vi "Lab03_Correct.vi"() -> ()   [LabVIEW 2022 SP3]
uses:
  <vilib>/numeric/Random Number (Range) DBL.vi
panel:
  out "Phase":dbl
  out "Sum of Differences Graph":cluster{dbl[], dbl[]}(graph)
  out "Sum of Difference Array":dbl[](array[numeric])
  out "Noisy Signal":dbl[][](graph)
  in  "# of Periods":dbl
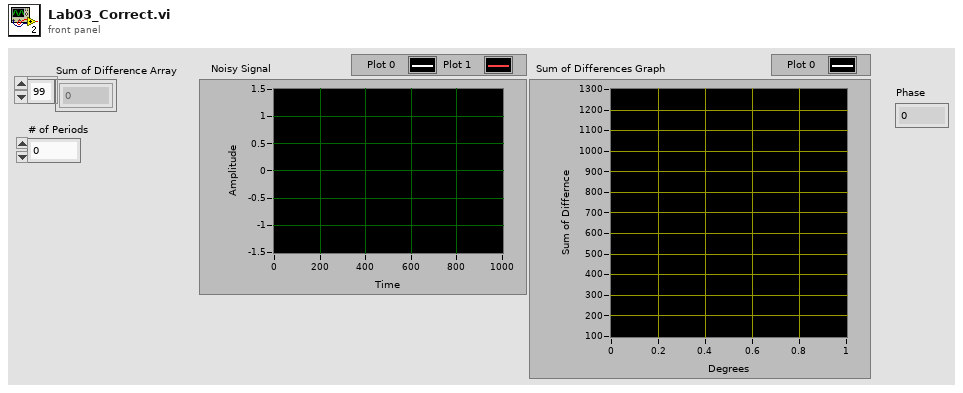
[diagram p1: front panel]
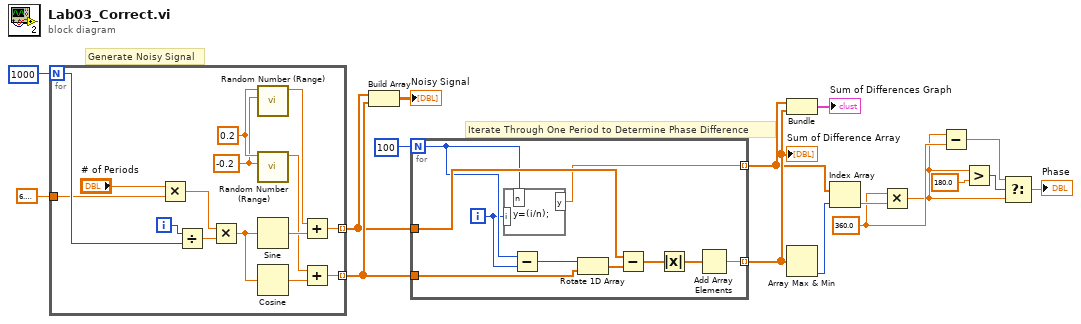
[diagram p0: block diagram]
diagram:
  w4 = 360.0 ("x")
  # "Iterate Through One Period to Determine Phase Difference"
  # "Generate Noisy Signal"
  n1 = for {
    N: 1000 -> [w22]
    tunnel: [w24] -> w14 mode=indexing
    tunnel: [w21] -> w15 mode=indexing
    tunnel: 6.283185307179586 -> [w18]
    i -> [w23]
    w31 = -0.2 ("lower bound (0)")
    w32 = 0.2 ("upper bound (100)")
    n2 = Multiply(x="# of Periods", y=w18) -> (x*y=w28:dbl)
    n3 = Divide(x=w23, y=w22) -> (x/y=w29:dbl)
    n4 = Multiply(x=w28, y=w29) -> (x*y=w27:dbl)
    n5 = call-poly <vilib>:"Random Number (Range).vi"("lower bound (0)"=w31, "upper bound (100)"=w32) -> ("number"=w20:dbl)  [unwired: 9 in]
    n6 = call-poly <vilib>:"Random Number (Range).vi"("lower bound (0)"=w31, "upper bound (100)"=w32) -> ("number"=w19:dbl)  [unwired: 9 in]
    n7 = Sine(x=w27) -> (sin(x)=w25:dbl)
    n8 = Cosine(x=w27) -> (cos(x)=w26:dbl)
    n9 = Add(x=w20, y=w25) -> (x+y=w24:dbl)
    n10 = Add(x=w19, y=w26) -> (x+y=w21:dbl)
  }
  n11 = Build Array(w14, w15) -> (→"Noisy Signal":dbl[][])
  n12 = for {
    N: 100 -> [w39]
    tunnel: w15 -> [w41]
    tunnel: w14 -> [w42]
    tunnel: [w33] -> w9 mode=indexing
    tunnel: [w34] -> w10 mode=indexing
    i -> [w37]
    n13 = formula code="y=(i/n);"("n"=w39, "i"=w37) -> ("y"=w33:dbl)
    n14 = Subtract(x=w39, y=w37) -> (x-y=w38:i32)
    n15 = Rotate 1D Array(1:w41, 2:w38) -> (0:w40:dbl[])
    n16 = Subtract(x=w42, y=w40) -> (x-y=w36:dbl[])
    n17 = Absolute Value(x=w36) -> (abs(x)=w35:dbl[])
    n18 = Add Array Elements(numeric array=w35) -> (sum=w34:dbl)
  }
  "Sum of Difference Array" <- w10
  n19 = Bundle(w9, w10) -> (→"Sum of Differences Graph":cluster{dbl[], dbl[]})  [unwired: 1 in]
  n20 = Array Max & Min(array=w10) -> (min index (indices)=w8:i32)  [unwired: 3 out]
  n21 = Index Array(array=w9, index=w8) -> (element=w7:dbl)
  n22 = Multiply(x=w4, y=w7) -> (x*y=w2:dbl)
  n23 = Subtract(x=w2, y=w4) -> (x-y=w3:dbl)
  n24 = Greater?(x=w2, y=180.0) -> (0:w5:bool)
  n25 = Select(t=w3, s=w5, f=w2) -> (s? t:f=→"Phase":dbl)
